vi "MK4DueReturnState.vi"(6 "error IN":errorcluster, 8 "String IN":string) -> (0 "error out":errorcluster, 1 "Return State 2":T1=enum."Echo", 3 "output cluster":T2)   [LabVIEW 2017]
uses:
  controls/STATE_MK4DUERETURNSTATE.ctl
  controls/state_board_control.ctl
panel:
  out "offset past match":i32
  out "String":string
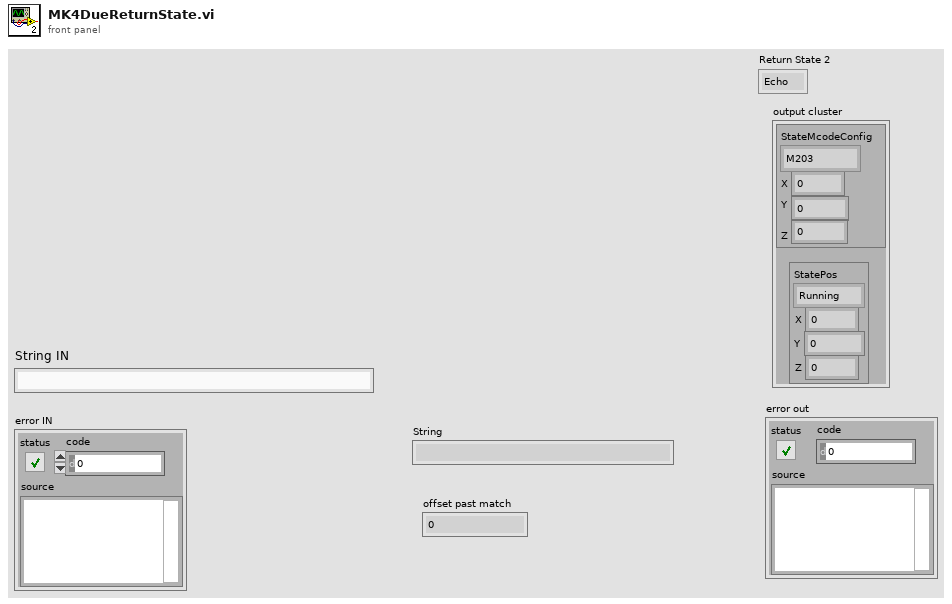
[diagram p1: front panel]
types:
  T1 = typedef "STATE_MK4DUERETURNSTATE.ctl" = enum16{"Pos", "Config", "Echo", "OK", "Step", "Error"}
  T2 = cluster{"OUTCONFIG":cluster{"StateMcodeConfig":enum16{"M203", "M201", "M92", "M3001"}, "X":dbl, "Y":dbl, "Z":dbl}, "outPOS":cluster{"StatePos":enum16{"Running", "Waiting", "Pos", "IDLE"}, "X":dbl, "Z":dbl, "Y":dbl}}
  T3 = cluster{"CODE_SETTING":cluster{"StateMcodeConfig":enum16{"M203", "M201", "M92", "M3001"}, dbl, dbl, dbl}, "CODE_VITRI":cluster{"Enum":enum16{"Running", "Waiting", "Pos", "IDLE"}, dbl, dbl, dbl}}
  T4 = typedef "state_board_control.ctl" = enum16{"Running", "Waiting", "Pos", "IDLE"}
  T5 = cluster{"StateMcodeConfig":enum16{"M203", "M201", "M92", "M3001"}, dbl, dbl, dbl}
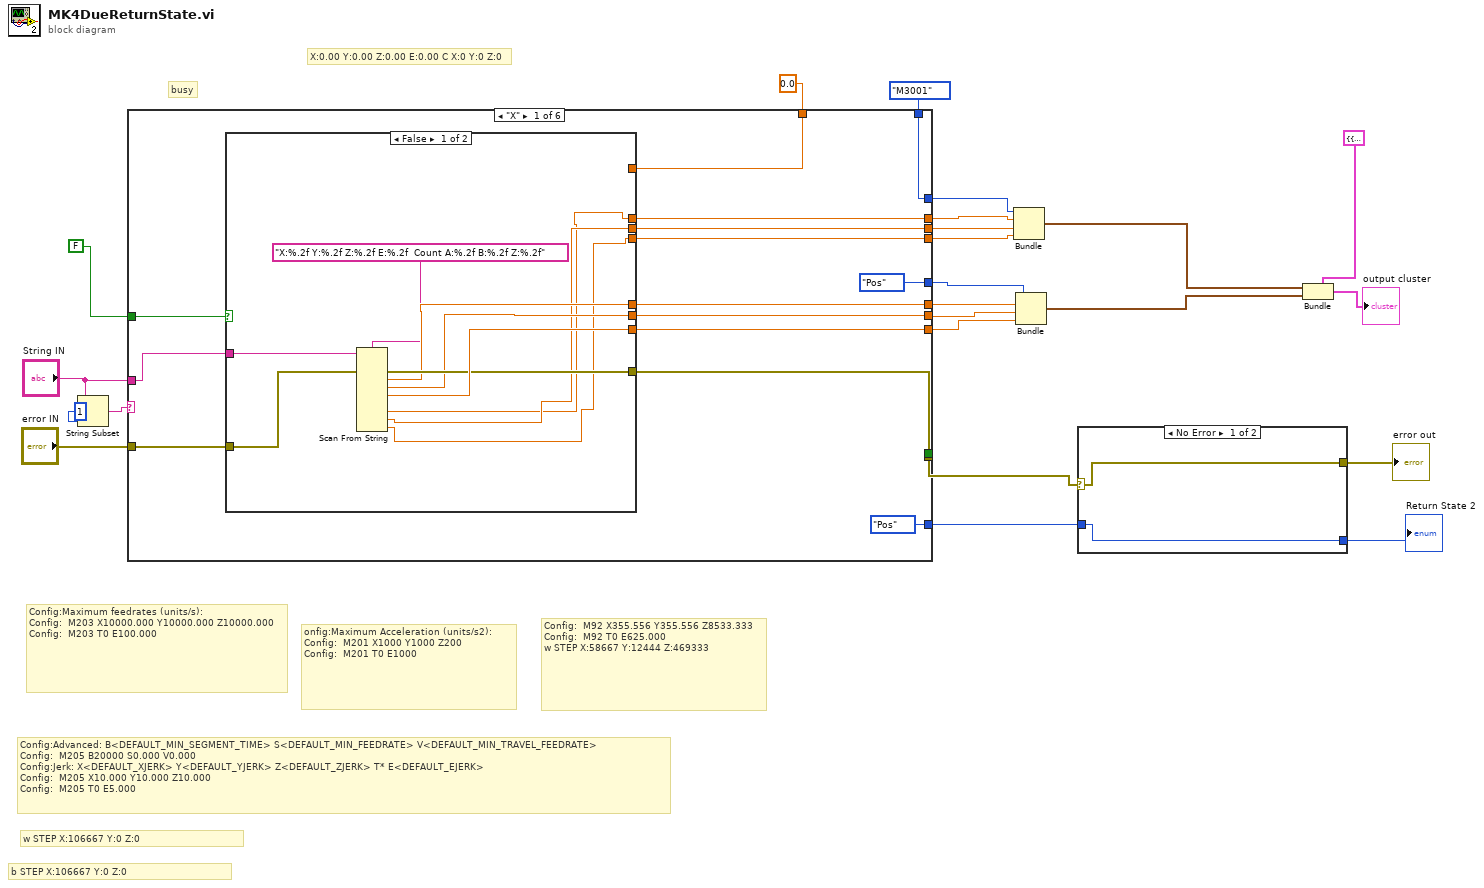
[diagram p0: block diagram]
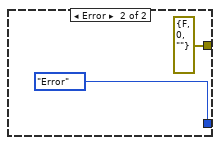
[diagram p2: hidden frame]
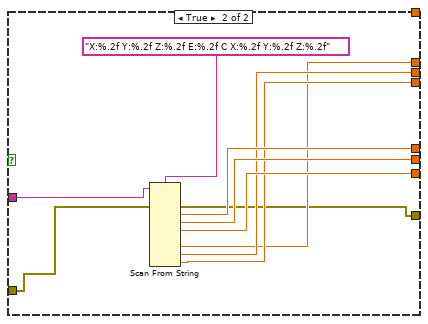
[diagram p3: hidden frame]
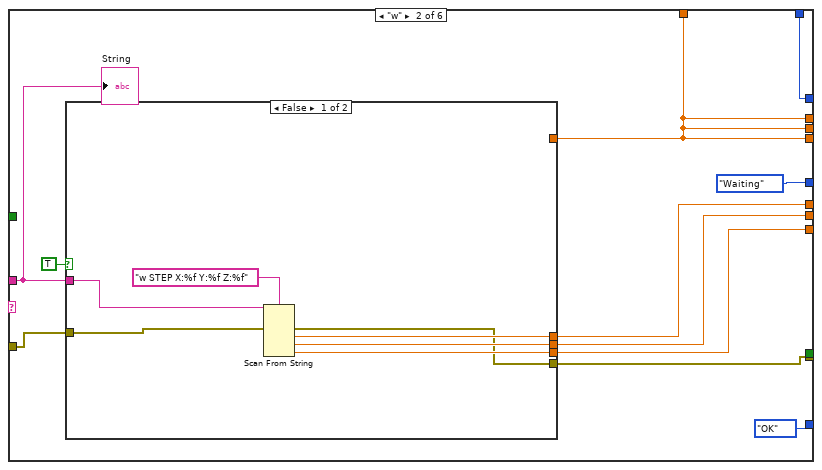
[diagram p4: hidden frame]
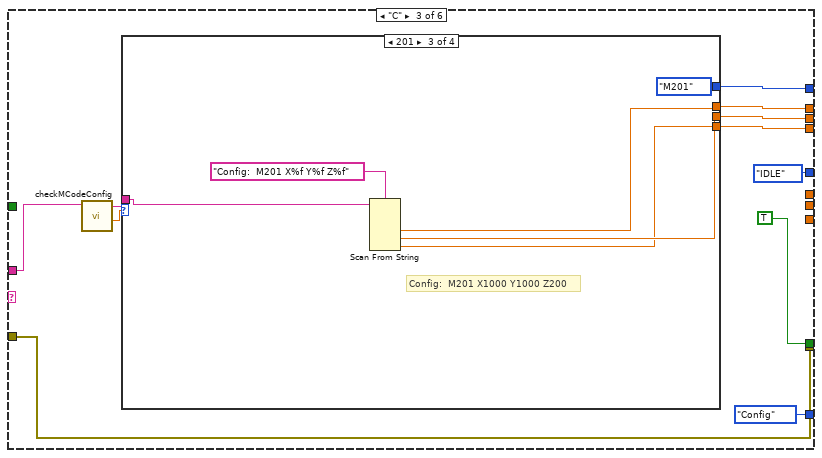
[diagram p6: hidden frame]
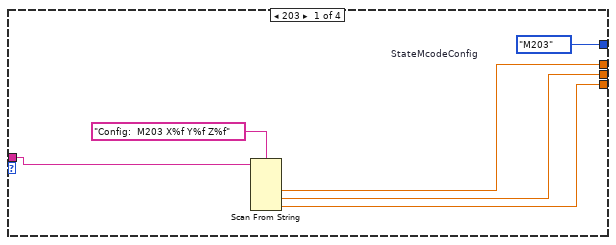
[diagram p7: hidden frame]
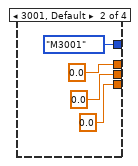
[diagram p8: hidden frame]
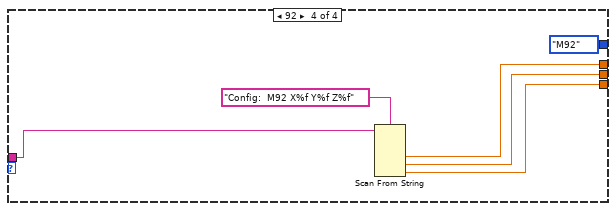
[diagram p9: hidden frame]
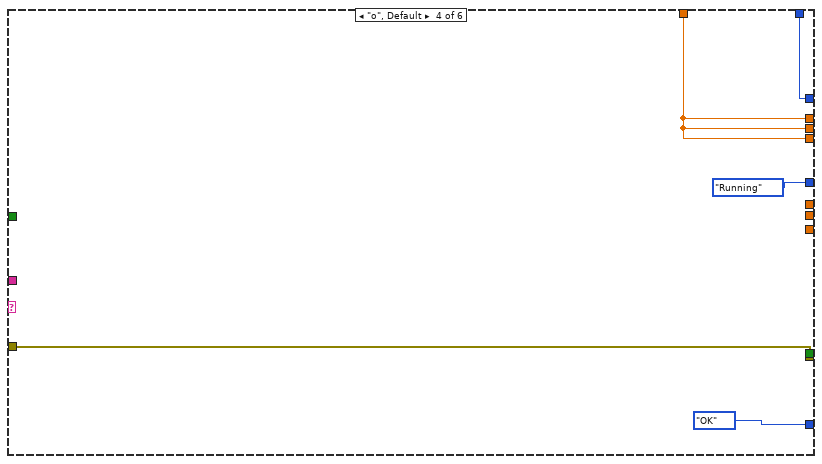
[diagram p10: hidden frame]
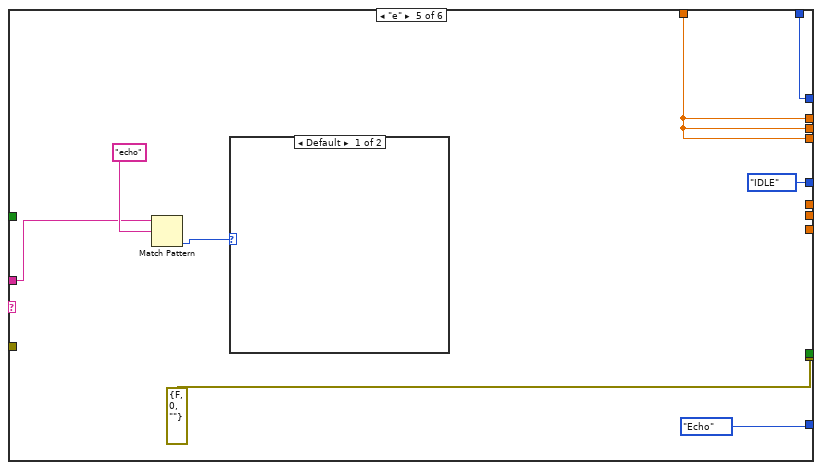
[diagram p11: hidden frame]
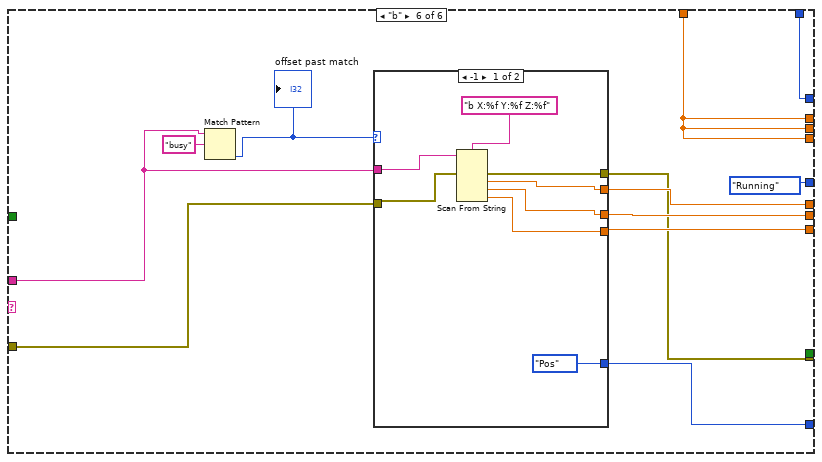
[diagram p13: hidden frame]
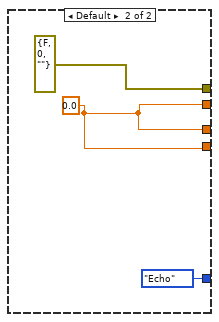
[diagram p14: hidden frame]
diagram:
  # "X:0.00 Y:0.00 Z:0.00 E:0.00 C X:0 Y:0 Z:0"
  # "busy"
  # "b STEP X:106667 Y:0 Z:0"
  # "Config:Advanced: B<DEFAULT_MIN_SEGMENT_TIME> S<DEFAULT_MIN_FEEDRATE> V<DEFAULT_MIN_TRAVEL_FEEDRATE>\nConfig:  M205 B20000 S0.000 V0.000\nConfig:Jerk: X<DEFAULT_XJERK> Y<DEFAULT_YJERK> Z<DEFAULT_ZJERK> T* E<DEFAULT_EJERK>\nConfig:  M205 X10.000 Y10.000 Z10.000\nConfig:  M205 T0 E5.000"
  # "Config:  M92 X355.556 Y355.556 Z8533.333\nConfig:  M92 T0 E625.000\nw STEP X:58667 Y:12444 Z:469333"
  # "onfig:Maximum Acceleration (units/s2):\nConfig:  M201 X1000 Y1000 Z200\nConfig:  M201 T0 E1000"
  # "Config:Maximum feedrates (units/s):\nConfig:  M203 X10000.000 Y10000.000 Z10000.000\nConfig:  M203 T0 E100.000"
  # "w STEP X:106667 Y:0 Z:0"
  n1 = String Subset(string="String IN", length (rest)=1 ("length (rest)")) -> (substring=w2:string)  [unwired: 1 in]
  n2 = case shown="\"X\"" w2 {
    tunnel: [state_board_control."Pos" ("Enum") enum16{"Running", "Waiting", "Pos", "IDLE"}."Waiting" ("Enum") enum16{"Running", "Waiting", "Pos", "IDLE"}."IDLE" ("Enum") enum16{"Running", "Waiting", "Pos", "IDLE"}."Running" ("Enum") enum16{"Running", "Waiting", "Pos", "IDLE"}."IDLE" ("Enum") enum16{"Running", "Waiting", "Pos", "IDLE"}."Running" ("Enum")] -> w22
    tunnel: [w32 w67 _ _ _ w129] -> w13
    tunnel: [w31 w66 _ _ _ w130] -> w12
    tunnel: [w37 w64 _ _ _ w131] -> w14
    tunnel: "error IN" -> [w36 w68 w88 w114 _ w127]
    tunnel: [w35 w62 w88 w114 errorcluster {"status"=FALSE, "code"=0, "source"=""} ("error IO") w128] -> w6
    tunnel: [w26 w59 w84 w112 w121 w135] -> w9
    tunnel: [w27 w59 w83 w112 w121 w135] -> w10
    tunnel: [w28 w59 w82 w112 w121 w135] -> w11
    tunnel: [w33 w65 w81 w113 w120 w126] -> w8
    tunnel: enum16{"M203", "M201", "M92", "M3001"}."M3001" ("StateMcodeConfig") -> [w33 w65 _ w113 w120 w126]
    tunnel: 0.0 -> [w25 w59 _ w112 w121 w135]
    tunnel: [_ _ TRUE ("Status") _ _ _] -> _
    tunnel: [STATE_MK4DUERETURNSTATE."Pos" ("Return State") STATE_MK4DUERETURNSTATE."OK" ("Return State") STATE_MK4DUERETURNSTATE."Config" ("Return State") STATE_MK4DUERETURNSTATE."OK" ("Return State") STATE_MK4DUERETURNSTATE."Echo" ("Return State") w125] -> w4
    tunnel: "String IN" -> [w29 w60 w78 _ w117 w124]
    tunnel: FALSE -> [w24 _ _ _ _ _]
    frame "X" {
      n3 = case shown="False" w24 {
        tunnel: [w47 w53] -> w37
        tunnel: w36 -> [w46 w49]
        tunnel: [w45 w48] -> w35
        tunnel: [w44 w55] -> w32
        tunnel: [w43 w54] -> w31
        tunnel: w29 -> [w42 w56]
        tunnel: [w40 w52] -> w28
        tunnel: [w39 w51] -> w27
        tunnel: [w38 w50] -> w26
        tunnel: w25 -> [_ _]
        frame False {
          n4 = Scan From String(format string="X:%.2f Y:%.2f Z:%.2f E:%.2f  Count A:%.2f B:%.2f Z:%.2f", input string=w42, error in=w46) -> (error out=w45:errorcluster, output 1=w44:dbl, output 2=w43:dbl, output 3=w47:dbl, output 5=w38:dbl, output 6=w39:dbl, output 7=w40:dbl)  [unwired: 9 in, 2 out]
        }
        frame True {
          n5 = Scan From String(format string="X:%.2f Y:%.2f Z:%.2f E:%.2f C X:%.2f Y:%.2f Z:%.2f", input string=w56, error in=w49) -> (error out=w48:errorcluster, output 1=w55:dbl, output 2=w54:dbl, output 3=w53:dbl, output 5=w50:dbl, output 6=w51:dbl, output 7=w52:dbl)  [unwired: 9 in, 2 out]
        }
      }
    }
    frame "w" {
      n6 = case shown="False" TRUE {
        tunnel: w68 -> [w74 w77]
        tunnel: [w73 w76] -> w67
        tunnel: [w72 w76] -> w66
        tunnel: [w71 w76] -> w64
        tunnel: [w70 w77] -> w62
        tunnel: w60 -> [w69 _]
        tunnel: w59 -> [_ w76]
        frame False {
          n7 = Scan From String(format string="w STEP X:%f Y:%f Z:%f", input string=w69, error in=w74) -> (error out=w70:errorcluster, output 1=w73:dbl, output 2=w72:dbl, output 3=w71:dbl)  [unwired: 4 in, 2 out]
        }
        frame True {
        }
      }
      "String" <- w60
    }
    frame "C" {
      n8 = call "checkMCodeConfig.vi"("INPUT"=w78) -> ("MCODE"=w86:dbl, "OUTPUT"=w85:string)  [unwired: 9 in]
      n9 = case shown="201" w86 {
        tunnel: w85 -> [w93 _ w103 w109]
        tunnel: [w92 0.0 w102 w108] -> w84
        tunnel: [w91 0.0 w101 w107] -> w83
        tunnel: [w90 0.0 w100 w106] -> w82
        tunnel: [w89 enum16{"M203", "M201", "M92", "M3001"}."M3001" ("StateMcodeConfig") enum16{"M203", "M201", "M92", "M3001"}."M201" ("StateMcodeConfig") enum16{"M203", "M201", "M92", "M3001"}."M92" ("StateMcodeConfig")] -> w81
        frame 203 {
          w89 = enum16{"M203", "M201", "M92", "M3001"}."M203"  # StateMcodeConfig
          n10 = Scan From String(format string="Config:  M203 X%f Y%f Z%f", input string=w93) -> (output 1=w92:dbl, output 2=w91:dbl, output 3=w90:dbl)  [unwired: 5 in, 3 out]
        }
        frame 3001, Default {
        }
        frame 201 {
          # "Config:  M201 X1000 Y1000 Z200"
          n11 = Scan From String(format string="Config:  M201 X%f Y%f Z%f", input string=w103) -> (output 1=w102:dbl, output 2=w101:dbl, output 3=w100:dbl)  [unwired: 5 in, 3 out]
        }
        frame 92 {
          n12 = Scan From String(format string="Config:  M92 X%f Y%f Z%f", input string=w109) -> (output 1=w108:dbl, output 2=w107:dbl, output 3=w106:dbl)  [unwired: 5 in, 3 out]
        }
      }
    }
    frame "o", Default {
    }
    frame "e" {
      n13 = Match Pattern(string=w117, regular expression="echo") -> (offset past match=w122:i32)  [unwired: 1 in, 3 out]
      n14 = case shown="Default" w122 {
        frame Default {
        }
        frame -1 {
        }
      }
    }
    frame "b" {
      n15 = Match Pattern(string=w124, regular expression="busy") -> (offset past match=w132:i32)  [unwired: 1 in, 3 out]
      "offset past match" <- w132
      n16 = case shown="-1" w132 {
        tunnel: w127 -> [w143 _]
        tunnel: [w142 errorcluster {"status"=FALSE, "code"=0, "source"=""} ("error IO")] -> w128
        tunnel: [w138 w145] -> w130
        tunnel: [w137 w145] -> w129
        tunnel: [w139 w145] -> w131
        tunnel: w124 -> [w141 _]
        tunnel: [STATE_MK4DUERETURNSTATE."Pos" ("Return State") STATE_MK4DUERETURNSTATE."Echo" ("Return State")] -> w125
        frame -1 {
          n17 = Scan From String(format string="b X:%f Y:%f Z:%f", input string=w141, error in=w143) -> (error out=w142:errorcluster, output 1=w137:dbl, output 2=w138:dbl, output 3=w139:dbl)  [unwired: 4 in, 2 out]
        }
        frame Default {
          w145 = 0.0
        }
      }
    }
  }
  n18 = Bundle("StateMcodeConfig"=w8, w9, w10, w11) -> (w17:T5)  [unwired: 1 in]
  n19 = Bundle("Enum"=w22, w13, w12, w14) -> (w18:cluster{"Enum":T4, dbl, dbl, dbl})  [unwired: 1 in]
  n20 = case shown="No Error" w6 {
    selector: w6 -> [w148 _]
    tunnel: [w148 errorcluster {"status"=FALSE, "code"=0, "source"=""} ("error IO")] -> w16
    tunnel: w4 -> [w147 _]
    tunnel: [w147 STATE_MK4DUERETURNSTATE."Error" ("Return State")] -> w5
    frame No Error {
    }
    frame Error {
    }
  }
  "error out" <- w16
  "Return State 2" <- w5
  n21 = Bundle(cluster=T3 {"CODE_SETTING"={"StateMcodeConfig"=enum."M203", 0.0, 0.0, 0.0}, "CODE_VITRI"={"Enum"=enum."Running", 0.0, 0.0, 0.0}}, "CODE_SETTING"=w17, "CODE_VITRI"=w18) -> (→"output cluster":T3)
